vi "Read UID.vi"(11 "Base Attributes in":refnum<class "Base Attributes.lvclass">) -> (2 "UID":string)   [LabVIEW 2020, in "jettl.lvlib" / "Base Attributes.lvlib" / "Base Attributes.lvclass"]
uses:
  Base Attributes.lvclass
  Base Attributes.lvclass/Base Attributes.ctl
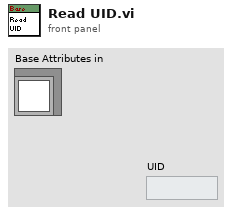
[diagram p1: front panel]
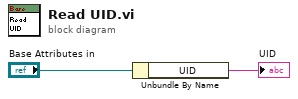
[diagram p0: block diagram]
diagram:
  n1 = Unbundle By Name("Base Attributes in") -> ("UID"=→"UID":string)
